vi "mqttCmdCreate.vi"(8 "error in (no error)":errorcluster, 10 "subscriptionInfo":T1[](array[typedef])) -> (0 "error out":errorcluster, 3 "mqttCmdSubscribe out":refnum<class "SubscribeMqttMsg.lvclass">)   [LabVIEW 2020, in "SubscribeMqttMsg.lvclass"]
uses:
  SubscribeMqttMsg.lvclass
  mqttTypedef/SubscribeData.ctl
  mqttTypedef/QosLevel.ctl
  SubscribeMqttMsg.lvclass/SubscribeMqttMsg.ctl
  BaseMqttMsg.lvclass
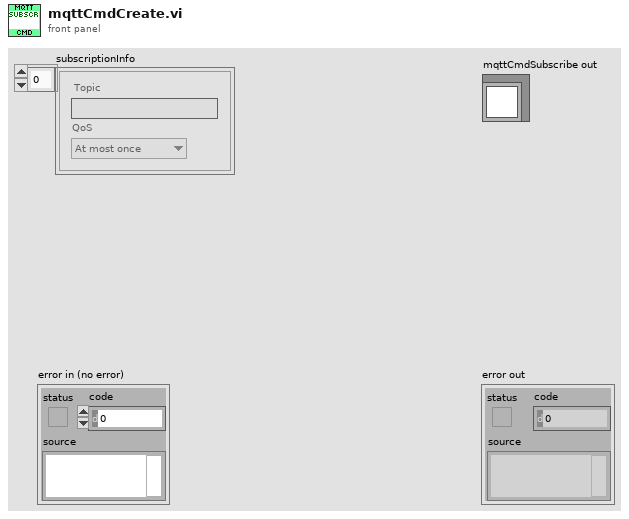
[diagram p1: front panel]
types:
  T1 = typedef "SubscribeMqttMsg.lvclass/SubscribeData.ctl" = cluster{"Topic":string, "QoS":T2}
  T2 = typedef "BaseMqttMsg.lvclass/QosLevel.ctl" = enum8{"At most once", "At least once", "Exactly once", "Reserved"}
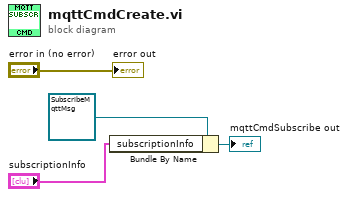
[diagram p0: block diagram]
diagram:
  n1 = Bundle By Name(cluster=refnum<class "SubscribeMqttMsg.lvclass"> refnum ("mqttCmdSubscribe in"), "subscriptionInfo"="subscriptionInfo") -> (→"mqttCmdSubscribe out":refnum<class "SubscribeMqttMsg.lvclass">)
  "error out" <- "error in (no error)"
